vi "CreateBrick.vi"(8 "error in (no error)":errorcluster, 11 "class data in":refnum<class "Brick.lvclass">) -> (0 "error out":errorcluster, 3 "class data out":refnum<class "Brick.lvclass">)   [LabVIEW 2010, in "Labricks.lvlib" / "Brick.lvclass"]
uses:
  Brick.lvclass
  <vilib>/picture/3D Picture Control/NI_3D Picture Control.lvlib
  RenderBase/SceneObject_class/SceneObject.lvclass
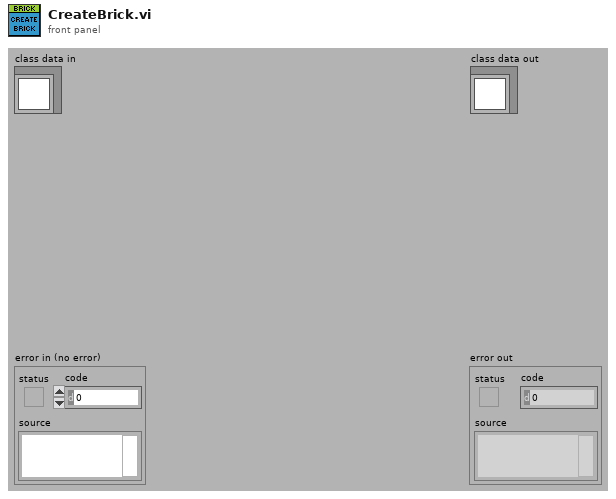
[diagram p1: front panel]
types:
  T1 = cluster{"number: 0 to 1":dbl, "number: 0 to 1":dbl, "number: 0 to 1":dbl, dbl}
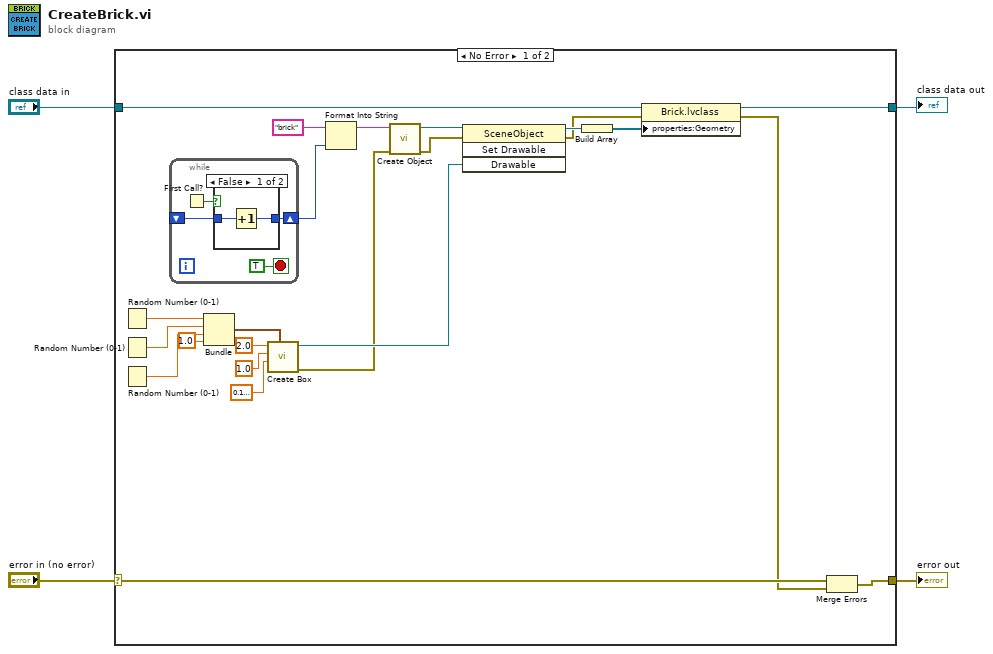
[diagram p0: block diagram]
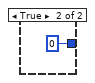
[diagram p2: hidden frame]
diagram:
  n1 = case shown="No Error" "error in (no error)" {
    selector: "error in (no error)" -> [w27 w36]
    tunnel: [w6 w36] -> w3
    tunnel: "class data in" -> [w26 w35]
    tunnel: [w22 w35] -> w1
    frame No Error {
      n2 = Random Number (0-1)() -> (number: 0 to 1=w15:dbl)
      n3 = Random Number (0-1)() -> (number: 0 to 1=w14:dbl)
      n4 = Random Number (0-1)() -> (number: 0 to 1=w13:dbl)
      n5 = while {
        shift-right: [w30] -> w16
        shift-left: _ -> [w29]
        stop <- TRUE stop-if-true
        n6 = First Call?() -> (First Call?: T/F=w28:bool)
        n7 = case shown="False" w28 {
          tunnel: [w33 0] -> w30
          tunnel: w29 -> [w32 _]
          frame False {
            n8 = Increment(x=w32) -> (x+1=w33:i32)
          }
          frame True {
          }
        }
      }
      n9 = Bundle("number: 0 to 1"=w15, "number: 0 to 1"=w14, "number: 0 to 1"=w13, 1.0) -> (w12:T1)  [unwired: 1 in]
      n10 = call <vilib>:"Create Box.vi"("Color"=w12, "Length Z"=sgl 0.1, "Length Y"=sgl 1.0, "Length X"=sgl 2.0 ("Radius")) -> ("error out"=w9:errorcluster, "New Box Refnum"=w25:refnum<vi>)  [unwired: 6 in]
      n11 = Format Into String(initial string="brick" ("Name"), w16) -> (resulting string=w17:string)  [unwired: 2 in, 1 out]
      n12 = call <vilib>:"Create Object.vi"("error in (no error)"=w9, "Name"=w17) -> ("error out"=w8:errorcluster, "Scene:New Object"=w23:refnum<vi>)  [unwired: 8 in]
      n13 = invoke class="SceneObject" method="Set Drawable"(reference=w23, error in=w8, "Drawable"=w25) -> (reference out=w21:refnum<vi>, error out=w7:errorcluster)  [unwired: 1 in, 2 out]
      n14 = Build Array(w21) -> (w10:refnum<vi>[])
      n15 = property class="Brick.lvclass"(reference=w26, error in=w7, "properties:Geometry"=w10) -> (reference out=w22:refnum<class "Brick.lvclass">, error out=w5:errorcluster)
      n16 = Merge Errors(w27, w5) -> (w6:errorcluster)
    }
    frame Error {
    }
  }
  "error out" <- w3
  "class data out" <- w1
